vi "Remove Image Padding.vi"(8 "error in (no error)":errorcluster, 11 "Image":T1) -> (0 "error out":errorcluster, 3 "Image Out":T1)   [LabVIEW 2020, in "G-Image.lvlib"]
doc: "Removes byte padding from image data, resulting from LabVIEW's image read functions.\n\nPadding is present at the end of each row in 8-bit images with an odd pixel width."
uses:
  G-Image.lvlib
  <vilib>/picture/picture.llb/imagedata.ctl
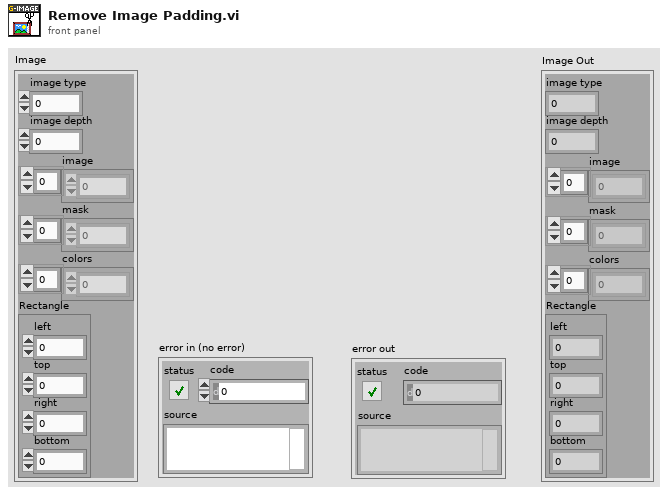
[diagram p1: front panel]
types:
  T1 = typedef "imagedata.ctl" = cluster{"image type":i32, "image depth":i32, "image":u8[], "mask":u8[], "colors":u32[], "Rectangle":cluster{"left":i16, "top":i16, "right":i16, "bottom":i16}}
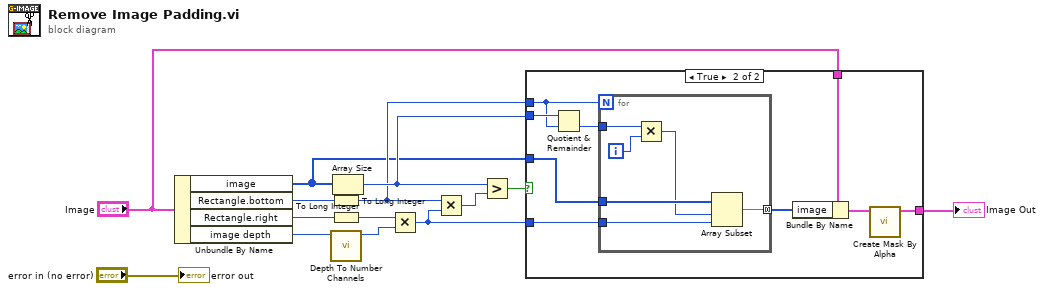
[diagram p0: block diagram]
diagram:
  n1 = Unbundle By Name("Image") -> ("image"=w3:u8[], "Rectangle.bottom"=w13:i16, "Rectangle.right"=w12:i16, "image depth"=w11:i32)
  n2 = To Long Integer(number=w13) -> (32bit integer=w6:i32)
  n3 = To Long Integer(number=w12) -> (32bit integer=w9:i32)
  n4 = call "Depth To Number Channels.vi"("Depth"=w11) -> ("Channels"=w10:i32)  [unwired: 10 in]
  n5 = Array Size(array=w3) -> (size(s)=w7:i32)
  n6 = Multiply(x=w9, y=w10) -> (x*y=w5:i32)
  n7 = Multiply(x=w6, y=w5) -> (x*y=w8:i32)
  n8 = Greater?(x=w7, y=w8) -> (0:w4:bool)
  n9 = case shown="True" w4 {
    tunnel: w7 -> [_ w24]
    tunnel: w6 -> [_ w23]
    tunnel: w5 -> [_ w22]
    tunnel: w3 -> [_ w20]
    tunnel: "Image" -> [w15 w17]
    tunnel: [w15 w16] -> w1
    frame False {
    }
    frame True {
      n10 = Quotient & Remainder(x=w24, y=w23) -> (floor(x/y)=w21:i32)  [unwired: 1 out]
      n11 = for {
        N: w23 -> [_]
        tunnel: w20 -> [w30]
        tunnel: w22 -> [w29]
        tunnel: w21 -> [w28]
        tunnel: [w25] -> w18 mode=concatenating
        i -> [w27]
        n12 = Multiply(x=w28, y=w27) -> (x*y=w26:i32)
        n13 = Array Subset(array=w30, index=w26, length=w29) -> (w25:u8[])
      }
      n14 = Bundle By Name(cluster=w17, "image"=w18) -> (w19:T1)
      n15 = call <vilib>:"Create Mask By Alpha.vi"("image data"=w19) -> ("masked image data"=w16:T1)  [unwired: 10 in]
    }
  }
  "Image Out" <- w1
  "error out" <- "error in (no error)"
